vi "Receive.vi"(11 "TEMPLATE Queue in":refnum<class "TEMPLATE Queue.lvclass">) -> (2 "Msg Strategy":refnum<class "Msg Strategy.lvclass">, 3 "TEMPLATE Queue out":refnum<class "TEMPLATE Queue.lvclass">)   [LabVIEW 2021, in "_Template.lvlib" / "Templates.lvlib" / "TEM Queue.lvlib" / "TEMPLATE Queue.lvclass"]
uses:
  TEMPLATE Queue.lvclass
  <vilib>/Nathan Davis/jettl/jettl/Msg Strategy/Msg Strategy.lvclass
  TEMPLATE Queue.lvclass/TEMPLATE Queue.ctl
  <vilib>/Nathan Davis/jettl/jettl/Queue/Queue.lvclass
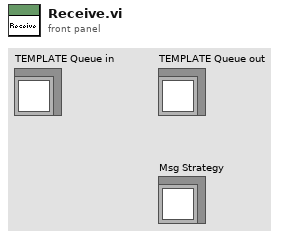
[diagram p1: front panel]
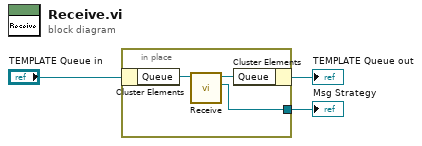
[diagram p0: block diagram]
diagram:
  n1 = in-place {
    in-place-border: [w4] -> w1
    n2 = in-place-cluster #1("TEMPLATE Queue in") -> ("Queue"=w6:refnum<class "Queue.lvclass">)
    n3 = call-dynamic "Receive.vi"("Queue in"=w6) -> ("Msg Strategy"=w4:refnum<class "Msg Strategy.lvclass">, "Queue out"=w5:refnum<class "Queue.lvclass">)  [unwired: 9 in]
    n4 = in-place-cluster #1("Queue"=w5) -> (→"TEMPLATE Queue out":refnum<class "TEMPLATE Queue.lvclass">)
  }
  "Msg Strategy" <- w1
